vi "Camera.vi"(0 "Camera in":refnum<class "Camera.lvclass">, 1 "Stop":bool, 4 "BCG Image Processing":T2={"Brightness"=128.0, "Contrast"=45.0, "Gamma"=1.0} {"Brightness" scale=0.0..400.0; "Contrast" scale=0.0..90.0; "Gamma" scale=0.005..5.0}, 5 "error in (no error)":errorcluster, 6 "Machine Vision":T4, 7 "Camera settings":T1={"Gamma"=1.0, "Gain"=7, "Sharpness"=0, "Contrast"=0.009999999999999995, "Exposure"=0.0004073180282999787} {"Exposure" min=0.000244140625 max=0.5 scale=0.0002..0.5; "Contrast" min=0.0 max=1.0 scale=0.001..1.0; "Sharpness" min=0 max=2 step=1 scale=0.0..2.0; "Gain" min=0 max=100 step=1 scale=0.1..100.0; "Gamma" min=0.01 max=10.0 scale=0.01..10.0}, 10 "Material":T3, 12 "Loop 0":bool, 13 "Override presets":bool) -> (11 "Radius (Real-World)":dbl, 14 "Camera out":refnum<class "Camera.lvclass">, 15 "Average Strength":dbl, 17 "Image":T5(plugin-control), 18 "Camera":dbl[](array[numeric]), 19 "error out":errorcluster)   [LabVIEW 2018, in "Camera.lvclass"]
uses:
  Camera.lvclass
  Machine Vision.ctl
  Material.ctl
  Image processing.ctl
  Camera settings.ctl
  <vilib>/vision/NI_Vision_Development_Module.lvlib
panel:
  out "Y":sgl
  out "X":sgl
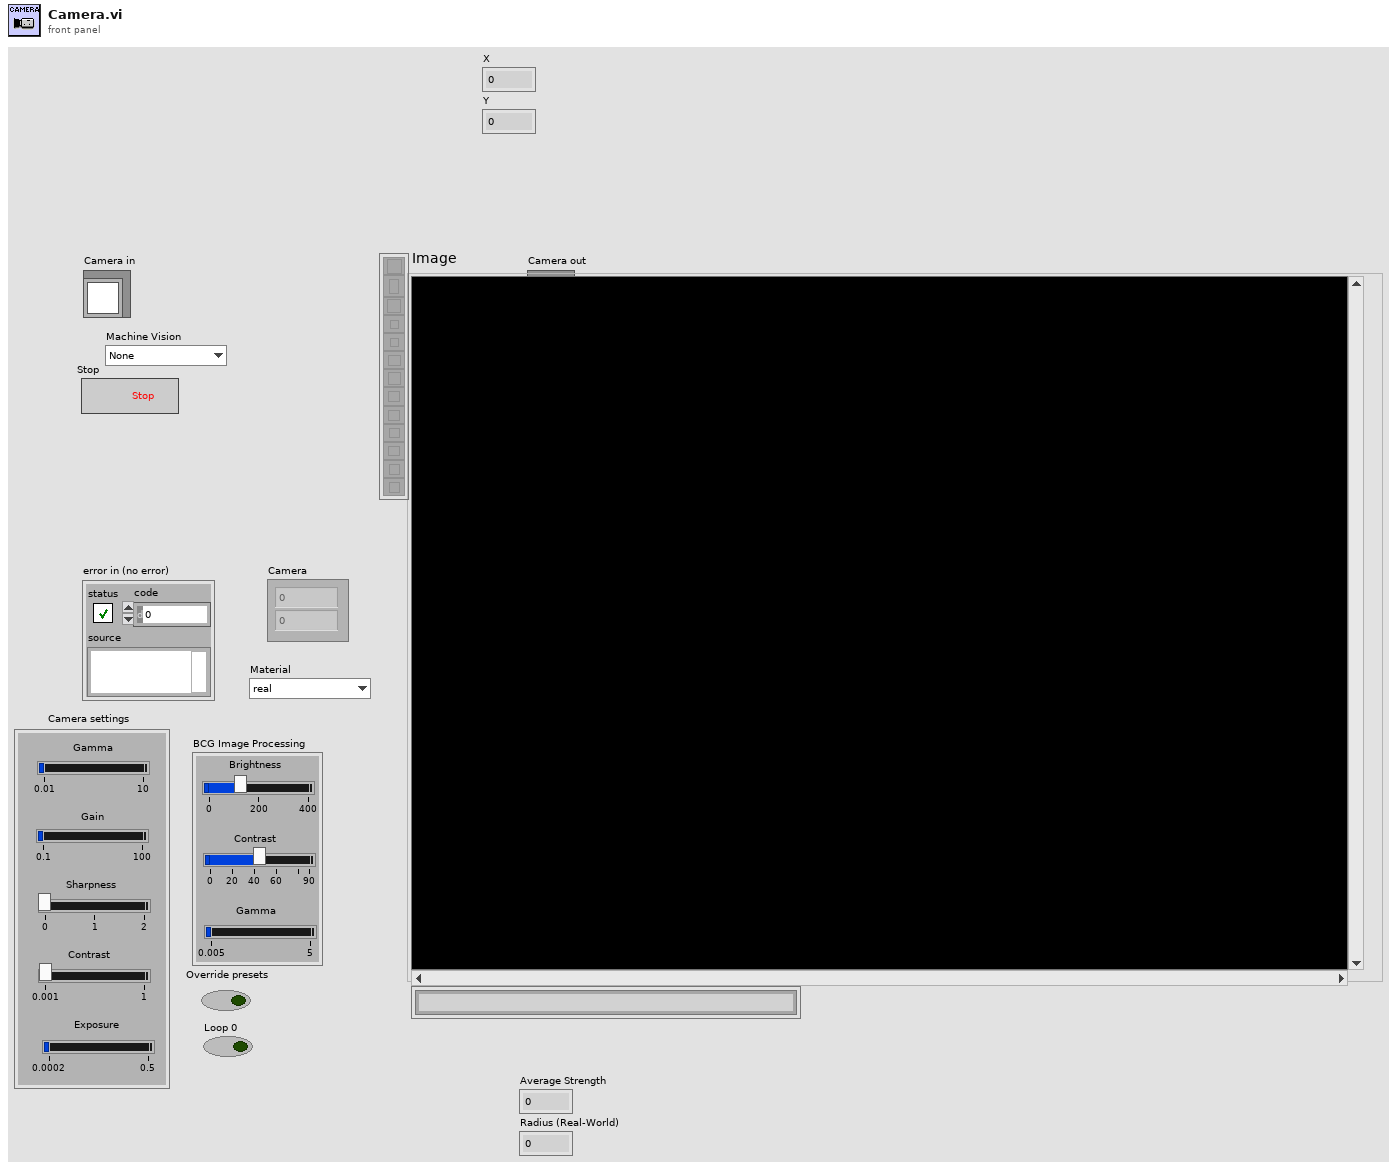
[diagram p1: front panel]
types:
  T1 = typedef "Camera.lvclass/Camera settings.ctl" = cluster{"Gamma":dbl, "Gain":i64, "Sharpness":i64, "Contrast":dbl, "Exposure":dbl}
  T2 = typedef "Camera.lvclass/Image processing.ctl" = cluster{"Brightness":sgl, "Contrast":sgl, "Gamma":sgl}
  T3 = typedef "Camera.lvclass/Material.ctl" = enum16{"real", "dummy", "PETG"}
  T4 = typedef "Camera.lvclass/Machine Vision.ctl" = enum16{"None", "Tray Fiducials", "HPK Silicon", "100um dot", "Hexaboard", "Corner (TL, BR)", "Corner (BL, TR)", "BP gold pad 1", "BP gold pad 2", "BP gold pad 3", "dummy sensor CH2", "dummy sensor CH7", "dummy sensor CH191", "dummy sensor CH197", "sensor box", "sensor circle", "PCB PETG CH2", "PCB PETG CH7", "PCB PETG CH191", "PCB PETG CH197"}
  T5 = typedef "IMAQ Image.ctl" = refnum<image>
  T6 = cluster{"Center (Pixels)":cluster{"X":sgl, "Y":sgl}, "Radius (Pixels)":dbl, "Center (Real-World)":cluster{"X":sgl, "Y":sgl}, "Radius (Real-World)":dbl, "Roundness (Real-World)":dbl, "Average Strength":dbl, "Average SNR (dB)":dbl}
  T7 = typedef "Edge New.ctl" = cluster{"Location (Pixel)":cluster{"X":sgl, "Y":sgl}, "Location (Real-World)":cluster{"X":sgl, "Y":sgl}, "Distance (Pixel)":dbl, "Distance (Real-World)":dbl, "Strength":dbl, "Noise":dbl, "Rising?":bool}
  T8 = cluster{"output string":sgl, "output string":sgl}
  T9 = typedef "ROI Descriptor" = cluster{"Global Rectangle":i32[], "Contours":cluster{"ID":enum32{"External", "Internal"}, "Type":u32, "Coordinates":i32[]}[]}
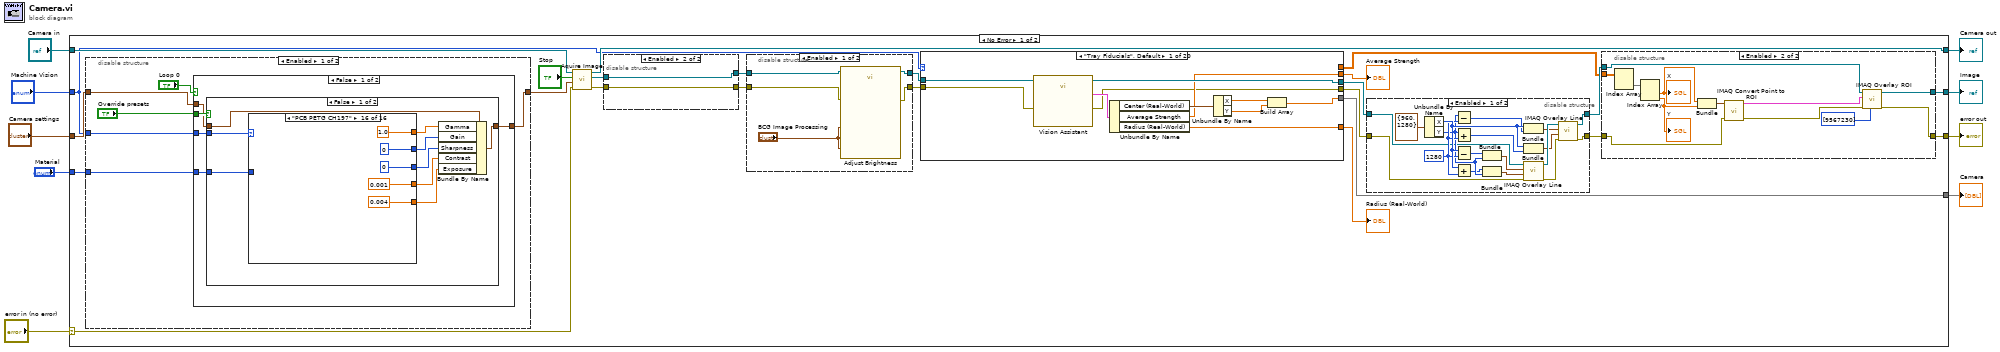
[diagram p0: block diagram]
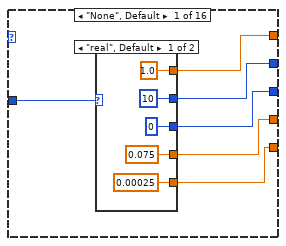
[diagram p5: hidden frame]
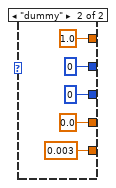
[diagram p6: hidden frame]
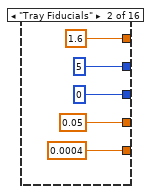
[diagram p7: hidden frame]
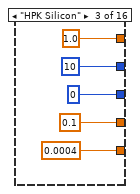
[diagram p8: hidden frame]
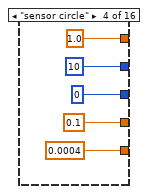
[diagram p9: hidden frame]
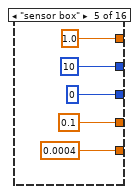
[diagram p10: hidden frame]
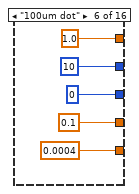
[diagram p11: hidden frame]
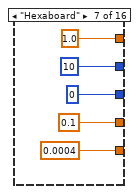
[diagram p12: hidden frame]
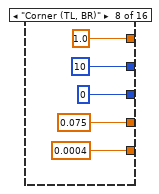
[diagram p13: hidden frame]
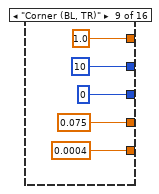
[diagram p14: hidden frame]
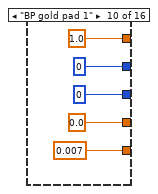
[diagram p15: hidden frame]
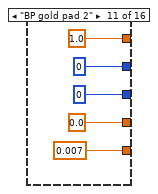
[diagram p16: hidden frame]
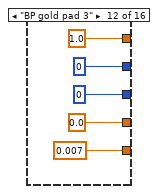
[diagram p17: hidden frame]
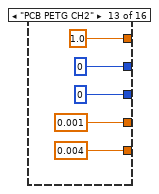
[diagram p18: hidden frame]
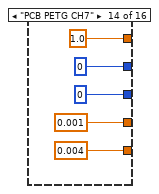
[diagram p19: hidden frame]
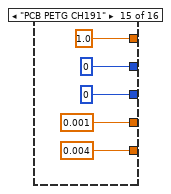
[diagram p20: hidden frame]
diagram:
  n1 = case shown="No Error" "error in (no error)" {
    selector: "error in (no error)" -> [w16 w391]
    tunnel: [w10 w391] -> w8
    tunnel: [w31 w390] -> w7
    tunnel: "Camera in" -> [w32 w390]
    tunnel: [w30 _] -> w5
    tunnel: [w20 _] -> w4
    tunnel: "Machine Vision" -> [w26 _]
    tunnel: "Camera settings" -> [w27 _]
    tunnel: "Material" -> [w25 _]
    frame No Error {
      n2 = disable-structure shown="Enabled" {
        disable-tunnel: w26 -> [w80 _]
        disable-tunnel: w27 -> [w79 w194]
        disable-tunnel: [w78 w194] -> w28
        disable-tunnel: w25 -> [w75 _]
        frame Enabled {
          n3 = case shown="False" "Loop 0" {
            tunnel: "Override presets" -> [w85 _]
            tunnel: w80 -> [w84 _]
            tunnel: w79 -> [w83 w193]
            tunnel: [w82 w192] -> w78
            tunnel: w75 -> [w81 _]
            frame False {
              n4 = case shown="False" w85 {
                tunnel: w84 -> [w94 _]
                tunnel: w83 -> [w93 w186]
                tunnel: [w87 w186] -> w82
                tunnel: w81 -> [w86 _]
                frame False {
                  n5 = case shown="\"PCB PETG CH197\"" w94 {
                    tunnel: [w99 1.6 ("Gamma::Value") 1.0 ("Gamma::Value") 1.0 ("Gamma::Value") 1.0 ("Gamma::Value") 1.0 ("Gamma::Value") 1.0 ("Gamma::Value") 1.0 ("Gamma::Value") 1.0 ("Gamma::Value") 1.0 ("Gamma::Value") 1.0 ("Gamma::Value") 1.0 ("Gamma::Value") 1.0 ("Gamma::Value") 1.0 ("Gamma::Value") 1.0 ("Gamma::Value") 1.0 ("Gamma::Value")] -> w92
                    tunnel: [w95 i64 5 ("Gain::Value") i64 10 ("Gain::Value") i64 10 ("Gain::Value") i64 10 ("Gain::Value") i64 10 ("Gain::Value") i64 10 ("Gain::Value") i64 10 ("Gain::Value") i64 10 ("Gain::Value") i64 0 ("Gain::Value") i64 0 ("Gain::Value") i64 0 ("Gain::Value") i64 0 ("Gain::Value") i64 0 ("Gain::Value") i64 0 ("Gain::Value") i64 0 ("Gain::Value")] -> w91
                    tunnel: [w96 i64 0 ("Sharpness::Value") i64 0 ("Sharpness::Value") i64 0 ("Sharpness::Value") i64 0 ("Sharpness::Value") i64 0 ("Sharpness::Value") i64 0 ("Sharpness::Value") i64 0 ("Sharpness::Value") i64 0 ("Sharpness::Value") i64 0 ("Sharpness::Value") i64 0 ("Sharpness::Value") i64 0 ("Sharpness::Value") i64 0 ("Sharpness::Value") i64 0 ("Sharpness::Value") i64 0 ("Sharpness::Value") i64 0 ("Sharpness::Value")] -> w90
                    tunnel: [w97 0.05 ("Contrast::Value") 0.1 ("Contrast::Value") 0.1 ("Contrast::Value") 0.1 ("Contrast::Value") 0.1 ("Contrast::Value") 0.1 ("Contrast::Value") 0.075 ("Contrast::Value") 0.075 ("Contrast::Value") 0.0 ("Contrast::Value") 0.0 ("Contrast::Value") 0.0 ("Contrast::Value") 0.001 ("Contrast::Value") 0.001 ("Contrast::Value") 0.001 ("Contrast::Value") 0.001 ("Contrast::Value")] -> w89
                    tunnel: [w98 0.0004 ("Exposure::Value") 0.0004 ("Exposure::Value") 0.0004 ("Exposure::Value") 0.0004 ("Exposure::Value") 0.0004 ("Exposure::Value") 0.0004 ("Exposure::Value") 0.0004 ("Exposure::Value") 0.0004 ("Exposure::Value") 0.007 ("Exposure::Value") 0.007 ("Exposure::Value") 0.007 ("Exposure::Value") 0.004 ("Exposure::Value") 0.004 ("Exposure::Value") 0.004 ("Exposure::Value") 0.004 ("Exposure::Value")] -> w88
                    tunnel: w86 -> [w100 _ _ _ _ _ _ _ _ _ _ _ _ _ _ _]
                    frame "None", Default {
                      n6 = case shown="\"real\", Default" w100 {
                        tunnel: [1.0 ("Gamma::Value") 1.0 ("Gamma::Value")] -> w99
                        tunnel: [0.00025 ("Exposure::Value") 0.003 ("Exposure::Value")] -> w98
                        tunnel: [0.075 ("Contrast::Value") 0.0 ("Contrast::Value")] -> w97
                        tunnel: [i64 0 ("Sharpness::Value") i64 0 ("Sharpness::Value")] -> w96
                        tunnel: [i64 10 ("Gain::Value") i64 0 ("Gain::Value")] -> w95
                        frame "real", Default {
                        }
                        frame "dummy" {
                        }
                      }
                    }
                    frame "Tray Fiducials" {
                    }
                    frame "HPK Silicon" {
                    }
                    frame "sensor circle" {
                    }
                    frame "sensor box" {
                    }
                    frame "100um dot" {
                    }
                    frame "Hexaboard" {
                    }
                    frame "Corner (TL, BR)" {
                    }
                    frame "Corner (BL, TR)" {
                    }
                    frame "BP gold pad 1" {
                    }
                    frame "BP gold pad 2" {
                    }
                    frame "BP gold pad 3" {
                    }
                    frame "PCB PETG CH2" {
                    }
                    frame "PCB PETG CH7" {
                    }
                    frame "PCB PETG CH191" {
                    }
                    frame "PCB PETG CH197" {
                    }
                  }
                  n7 = Bundle By Name(cluster=w93, "Gamma"=w92, "Gain"=w91, "Sharpness"=w90, "Contrast"=w89, "Exposure"=w88) -> (w87:T1)
                }
                frame True {
                }
              }
            }
            frame True {
              n8 = Bundle By Name(cluster=w193, "Gamma"=0.01, "Gain"=i64 0, "Sharpness"=i64 0, "Contrast"=0.0, "Exposure"=0.000249) -> (w192:T1)
            }
          }
        }
        frame Disabled {
        }
      }
      n9 = call-dynamic "Aquire Image.vi"("error in (no error)"=w16, "Cluster"=w28, "Stop"="Stop", "Camera in"=w32) -> ("error out"=w15:errorcluster, "Image Out"=w29:T5, "Camera out"=w31:refnum<class "Camera.lvclass">)  [unwired: 5 in]
      n10 = disable-structure shown="Enabled" {
        disable-tunnel: w29 -> [w201 w204]
        disable-tunnel: [w200 w204] -> w24
        disable-tunnel: w15 -> [w197 w203]
        disable-tunnel: [w195 w203] -> w14
        frame Disabled {
          w199 = u32 1 items=["Horizontal", "Vertical", "Central", "1st Diagonal", "2nd Diagonal"] ("Type of Symmetry")
          n11 = call "IMAQ Rotate"("error in (no error)"=w197, "Angle (degrees)"=270, "Image Src"=w201) -> ("error out"=w196:errorcluster, "Image Dst Out"=w198:T5)  [unwired: 7 in]
          n12 = call "IMAQ Symmetry"("error in (no error)"=w196, "Type of Symmetry"=w199, "Image Src"=w198) -> ("error out"=w195:errorcluster, "Image Dst Out"=w200:T5)  [unwired: 2 in]
        }
        frame Enabled {
        }
      }
      n13 = disable-structure shown="Enabled" {
        disable-tunnel: w24 -> [w72 w73]
        disable-tunnel: [w70 w73] -> w23
        disable-tunnel: w14 -> [w69 w74]
        disable-tunnel: [w68 w74] -> w13
        frame Enabled {
          n14 = call "Adjust Brightness"("Image In"=w72, "Red BCG Values (Brightness 1)"="BCG Image Processing", "Green BCG Values (Brightness 1)"="BCG Image Processing", "Blue BCG Values (Brightness 1)"="BCG Image Processing", "error in"=w69) -> ("Image Out"=w70:T5, "error out"=w68:errorcluster)  [unwired: 21 in]
        }
        frame Disabled {
        }
      }
      n15 = case shown="\"Tray Fiducials\", Default" w26 {
        tunnel: [w209 w219 w227 w238 w246 w254 w262 w270 w278 w287 w298 w304 w317 w323 w335 w347 w358 w366 w374 w382] -> w30
        tunnel: [w211 w221 w228 w240 w248 w256 w264 w272 w280 w288 w299 w310 w318 w327 w339 w351 w364 w372 w380 w388] -> w22
        tunnel: w23 -> [w212 w221 w226 w237 w245 w253 w261 w269 w277 w285 w296 w309 w315 w328 w340 w352 w365 w373 w381 w389]
        tunnel: [w207 0.0 ("Radius (Real-World)") w224 0.0 ("Radius (Real-World)") 0.0 ("Radius (Real-World)") 0.0 ("Radius (Real-World)") 0.0 ("Radius (Real-World)") 0.0 ("Radius (Real-World)") 0.0 ("Radius (Real-World)") w284 w295 0.0 ("Radius (Real-World)") w314 0.0 ("Radius (Real-World)") 0.0 ("Radius (Real-World)") 0.0 ("Radius (Real-World)") 0.0 ("Radius (Real-World)") 0.0 ("Radius (Real-World)") 0.0 ("Radius (Real-World)") 0.0 ("Radius (Real-World)")] -> w19
        tunnel: [w208 0.0 ("Strength") w225 _ _ _ _ _ _ w283 w294 _ w313 w333 w345 w357 _ _ _ _] -> w18
        tunnel: [_ _ _ w236 w244 w252 w260 w268 w276 _ _ w306 _ _ _ _ w360 w368 w376 w384] -> w17
        tunnel: w13 -> [w206 w220 w222 w235 w243 w249 w257 w265 w273 w282 w293 w308 w312 w326 w338 w350 w363 w371 w379 w387]
        tunnel: [w205 w220 w223 w234 w242 w250 w258 w266 w274 w281 w292 w307 w311 w325 w337 w349 w362 w370 w378 w386] -> w12
        frame "Tray Fiducials", Default {
          n16 = call "Vision Assistant"("Image In"=w212, "error in"=w206) -> ("Image Out"=w211:T5, "Fitted Circle (Find Circular Edge 1)"=w210:T6, "error out"=w205:errorcluster)  [unwired: 23 in]
          n17 = Unbundle By Name(w210) -> ("Center (Real-World)"=w213:cluster{"X":sgl, "Y":sgl}, "Average Strength"=w208:dbl, "Radius (Real-World)"=w207:dbl)
          n18 = Unbundle By Name(w213) -> ("X"=w215:sgl, "Y"=w214:sgl)
          n19 = Build Array(w215, w214) -> (w209:sgl[])
        }
        frame "None" {
          n20 = Initialize Array(0.0 ("element")) -> (w219:dbl[])  [unwired: 1 in]
        }
        frame "Hexaboard" {
          n21 = call "Vision Assistant2"("Image In"=w226, "error in"=w222) -> ("Image Out"=w228:T5, "Fitted Circle (Find Circular Edge 1)"=w230:T6, "error out"=w223:errorcluster)  [unwired: 23 in]
          n22 = Unbundle By Name(w230) -> ("Center (Real-World)"=w232:cluster{"X":sgl, "Y":sgl}, "Average Strength"=w225:dbl, "Radius (Real-World)"=w224:dbl)
          n23 = Unbundle By Name(w232) -> ("X"=w231:sgl, "Y"=w229:sgl)
          n24 = Build Array(w231, w229) -> (w227:sgl[])
        }
        frame "Corner (TL, BR)" {
          n25 = call "Vision Assistant3"("Image In"=w237, "error in"=w235) -> ("Image Out"=w240:T5, "error out"=w234:errorcluster, "Caliper Results (Top Left, Bottom Right)"=w236:sgl[][], "Calibrated Results (Top Left, Bottom Right)"=w239:sgl[][])  [unwired: 22 in]
          n26 = Index Array(array=w239) -> (element=w238:sgl[])  [unwired: 2 in]
        }
        frame "Corner (BL, TR)" {
          n27 = call "Vision Assistant4"("Image In"=w245, "error in"=w243) -> ("Image Out"=w248:T5, "error out"=w242:errorcluster, "Caliper Results (Bottom Left, Top Right)"=w244:sgl[][], "Calibrated Results (Bottom Left, Top Right)"=w247:sgl[][])  [unwired: 22 in]
          n28 = Index Array(array=w247) -> (element=w246:sgl[])  [unwired: 2 in]
        }
        frame "dummy sensor CH2" {
          n29 = call "Vision Assistant10"("Image In"=w253, "error in"=w249) -> ("Image Out"=w256:T5, "Caliper Results (Top Left, Bottom Right)"=w252:sgl[][], "Calibrated Results (Top Left, Bottom Right)"=w255:sgl[][], "error out"=w250:errorcluster)  [unwired: 22 in]
          n30 = Index Array(array=w255) -> (element=w254:sgl[])  [unwired: 2 in]
        }
        frame "dummy sensor CH7" {
          n31 = call "Vision Assistant11"("Image In"=w261, "error in"=w257) -> ("Image Out"=w264:T5, "Caliper Results (Top Left, Bottom Right)"=w260:sgl[][], "Calibrated Results (Top Left, Bottom Right)"=w263:sgl[][], "error out"=w258:errorcluster)  [unwired: 22 in]
          n32 = Index Array(array=w263) -> (element=w262:sgl[])  [unwired: 2 in]
        }
        frame "dummy sensor CH191" {
          n33 = call "Vision Assistant12"("Image In"=w269, "error in"=w265) -> ("Image Out"=w272:T5, "Caliper Results (Top Left, Bottom Right)"=w268:sgl[][], "Calibrated Results (Top Left, Bottom Right)"=w271:sgl[][], "error out"=w266:errorcluster)  [unwired: 22 in]
          n34 = Index Array(array=w271) -> (element=w270:sgl[])  [unwired: 2 in]
        }
        frame "dummy sensor CH197" {
          n35 = call "Vision Assistant13"("Image In"=w277, "error in"=w273) -> ("Image Out"=w280:T5, "Caliper Results (Top Left, Bottom Right)"=w276:sgl[][], "Calibrated Results (Top Left, Bottom Right)"=w279:sgl[][], "error out"=w274:errorcluster)  [unwired: 22 in]
          n36 = Index Array(array=w279) -> (element=w278:sgl[])  [unwired: 2 in]
        }
        frame "HPK Silicon" {
          n37 = call "Vision Assistant5"("Image In"=w285, "error in"=w282) -> ("Image Out"=w288:T5, "Fitted Circle (Find Circular Edge 1)"=w286:T6, "error out"=w281:errorcluster)  [unwired: 23 in]
          n38 = Unbundle By Name(w286) -> ("Center (Real-World)"=w291:cluster{"X":sgl, "Y":sgl}, "Average Strength"=w283:dbl, "Radius (Real-World)"=w284:dbl)
          n39 = Unbundle By Name(w291) -> ("X"=w290:sgl, "Y"=w289:sgl)
          n40 = Build Array(w290, w289) -> (w287:sgl[])
        }
        frame "sensor circle" {
          n41 = call "Vision Assistant14"("Image In"=w296, "error in"=w293) -> ("Image Out"=w299:T5, "Fitted Circle (Find Circular Edge 1)"=w297:T6, "error out"=w292:errorcluster)  [unwired: 23 in]
          n42 = Unbundle By Name(w297) -> ("Center (Real-World)"=w302:cluster{"X":sgl, "Y":sgl}, "Average Strength"=w294:dbl, "Radius (Real-World)"=w295:dbl)
          n43 = Unbundle By Name(w302) -> ("X"=w301:sgl, "Y"=w300:sgl)
          n44 = Build Array(w301, w300) -> (w298:sgl[])
        }
        frame "sensor box" {
          n45 = call "Vision Assistant15"("Image In"=w309, "error in"=w308) -> ("Image Out"=w310:T5, "Caliper Results (Caliper 1)"=w306:sgl[][], "Calibrated Results (Caliper 1)"=w305:sgl[][], "error out"=w307:errorcluster)  [unwired: 22 in]
          n46 = Index Array(array=w305) -> (element=w304:sgl[])  [unwired: 2 in]
        }
        frame "100um dot" {
          n47 = call "Vision Assistant6"("Image In"=w315, "error in"=w312) -> ("Image Out"=w318:T5, "Fitted Circle (Find Circular Edge 1)"=w316:T6, "error out"=w311:errorcluster)  [unwired: 23 in]
          n48 = Unbundle By Name(w316) -> ("Center (Real-World)"=w321:cluster{"X":sgl, "Y":sgl}, "Average Strength"=w313:dbl, "Radius (Real-World)"=w314:dbl)
          n49 = Unbundle By Name(w321) -> ("X"=w320:sgl, "Y"=w319:sgl)
          n50 = Build Array(w320, w319) -> (w317:sgl[])
        }
        frame "BP gold pad 1" {
          n51 = call "Vision Assistant7"("Image In"=w328, "error in"=w326) -> ("Image Out"=w327:T5, "Used Edges (Adv. Straight Edge 1)"=w332:cluster{"Edge Information":T7[]}[], "error out"=w325:errorcluster)  [unwired: 23 in]
          n52 = Index Array(array=w332) -> (element=w331:cluster{"Edge Information":T7[]})  [unwired: 1 in]
          n53 = Unbundle By Name(w331) -> ("Edge Information"=w330:T7[])
          n54 = Index Array(array=w330) -> (element=w329:T7)  [unwired: 1 in]
          n55 = Unbundle(w329) -> ("Location (Real-World)"=w324:cluster{"X":sgl, "Y":sgl}, "Strength"=w333:dbl)  [unwired: 5 out]
          n56 = Cluster To Array(cluster=w324) -> (array=w323:sgl[])
        }
        frame "BP gold pad 2" {
          n57 = call "Vision Assistant8"("Image In"=w340, "error in"=w338) -> ("Image Out"=w339:T5, "Used Edges (Adv. Straight Edge 1)"=w344:cluster{"Edge Information":T7[]}[], "error out"=w337:errorcluster)  [unwired: 23 in]
          n58 = Index Array(array=w344) -> (element=w343:cluster{"Edge Information":T7[]})  [unwired: 1 in]
          n59 = Unbundle By Name(w343) -> ("Edge Information"=w342:T7[])
          n60 = Index Array(array=w342) -> (element=w341:T7)  [unwired: 1 in]
          n61 = Unbundle(w341) -> ("Location (Real-World)"=w336:cluster{"X":sgl, "Y":sgl}, "Strength"=w345:dbl)  [unwired: 5 out]
          n62 = Cluster To Array(cluster=w336) -> (array=w335:sgl[])
        }
        frame "BP gold pad 3" {
          n63 = call "Vision Assistant9"("Image In"=w352, "error in"=w350) -> ("Image Out"=w351:T5, "Used Edges (Adv. Straight Edge 1)"=w356:cluster{"Edge Information":T7[]}[], "error out"=w349:errorcluster)  [unwired: 23 in]
          n64 = Index Array(array=w356) -> (element=w355:cluster{"Edge Information":T7[]})  [unwired: 1 in]
          n65 = Unbundle By Name(w355) -> ("Edge Information"=w354:T7[])
          n66 = Index Array(array=w354) -> (element=w353:T7)  [unwired: 1 in]
          n67 = Unbundle(w353) -> ("Location (Real-World)"=w348:cluster{"X":sgl, "Y":sgl}, "Strength"=w357:dbl)  [unwired: 5 out]
          n68 = Cluster To Array(cluster=w348) -> (array=w347:sgl[])
        }
        frame "PCB PETG CH2" {
          n69 = call "Vision Assistant16"("Image In"=w365, "error in"=w363) -> ("Image Out"=w364:T5, "Caliper Results (Caliper 1)"=w360:sgl[][], "Calibrated Results (Caliper 1)"=w359:sgl[][], "error out"=w362:errorcluster)  [unwired: 22 in]
          n70 = Index Array(array=w359) -> (element=w358:sgl[])  [unwired: 2 in]
        }
        frame "PCB PETG CH7" {
          n71 = call "Vision Assistant17"("Image In"=w373, "error in"=w371) -> ("Image Out"=w372:T5, "Caliper Results (Caliper 1)"=w368:sgl[][], "Calibrated Results (Caliper 1)"=w367:sgl[][], "error out"=w370:errorcluster)  [unwired: 22 in]
          n72 = Index Array(array=w367) -> (element=w366:sgl[])  [unwired: 2 in]
        }
        frame "PCB PETG CH191" {
          n73 = call "Vision Assistant18"("Image In"=w381, "error in"=w379) -> ("Image Out"=w380:T5, "Caliper Results (Caliper 1)"=w376:sgl[][], "Calibrated Results (Caliper 1)"=w375:sgl[][], "error out"=w378:errorcluster)  [unwired: 22 in]
          n74 = Index Array(array=w375) -> (element=w374:sgl[])  [unwired: 2 in]
        }
        frame "PCB PETG CH197" {
          n75 = call "Vision Assistant19"("Image In"=w389, "error in"=w387) -> ("Image Out"=w388:T5, "Caliper Results (Caliper 1)"=w384:sgl[][], "Calibrated Results (Caliper 1)"=w383:sgl[][], "error out"=w386:errorcluster)  [unwired: 22 in]
          n76 = Index Array(array=w383) -> (element=w382:sgl[])  [unwired: 2 in]
        }
      }
      "Radius (Real-World)" <- w19
      "Average Strength" <- w18
      n77 = disable-structure shown="Enabled" {
        disable-tunnel: w22 -> [w52 w67]
        disable-tunnel: [w51 w67] -> w21
        disable-tunnel: w12 -> [w50 w66]
        disable-tunnel: [w48 w66] -> w11
        frame Enabled {
          w59 = 1280
          n78 = Unbundle By Name(cluster{"X":i32, "Y":i32} {"X"=960, "Y"=1280} ("Cross Hair coordinates")) -> ("X"=w62:i32, "Y"=w58:i32)
          n79 = Subtract(x=w58, y=w59) -> (x-y=w60:i32)
          n80 = Add(x=w58, y=w59) -> (x+y=w61:i32)
          n81 = Subtract(x=w62, y=w59) -> (x-y=w54:i32)
          n82 = Add(x=w62, y=w59) -> (x+y=w55:i32)
          n83 = Bundle(w54, "Y"=w58) -> (w57:cluster{i32, "Y":i32})  [unwired: 1 in]
          n84 = Bundle(w55, "Y"=w58) -> (w56:cluster{i32, "Y":i32})  [unwired: 1 in]
          n85 = Bundle("X"=w62, w60) -> (w63:cluster{"X":i32, i32})  [unwired: 1 in]
          n86 = Bundle("X"=w62, w61) -> (w64:cluster{"X":i32, i32})  [unwired: 1 in]
          n87 = call "IMAQ Overlay Line"("error in (no error)"=w50, "End Point"=w56, "Start Point"=w57, "Image"=w52) -> ("error out"=w49:errorcluster, "Image Out"=w65:T5)  [unwired: 6 in]
          n88 = call "IMAQ Overlay Line"("error in (no error)"=w49, "End Point"=w64, "Start Point"=w63, "Image"=w65) -> ("error out"=w48:errorcluster, "Image Out"=w51:T5)  [unwired: 6 in]
        }
        frame Disabled {
        }
      }
      n89 = disable-structure shown="Enabled" {
        disable-tunnel: [w35 w43] -> w20
        disable-tunnel: w21 -> [w35 w42]
        disable-tunnel: w17 -> [_ w41]
        disable-tunnel: w11 -> [w34 w38]
        disable-tunnel: [w34 w36] -> w10
        frame Disabled {
        }
        frame Enabled {
          n90 = Index Array(array=w41) -> (element=w40:sgl[])  [unwired: 2 in]
          n91 = Index Array(array=w40) -> (element #1=w44:sgl, element #2=w46:sgl)  [unwired: 2 in]
          "X" <- w44
          "Y" <- w46
          n92 = Bundle("output string"=w44, "output string"=w46) -> (w47:T8)  [unwired: 1 in]
          n93 = call "IMAQ Convert Point to ROI"("error in (no error)"=w38, "Point"=w47) -> ("error out"=w37:errorcluster, "ROI Descriptor"=w45:T9)  [unwired: 7 in]
          n94 = call "IMAQ Overlay ROI"("Colors (Green)"=u32[] [9567230], "error in (no error)"=w37, "ROI Descriptor"=w45, "Image"=w42) -> ("error out"=w36:errorcluster, "Image Out"=w43:T5)  [unwired: 6 in]
        }
      }
    }
    frame Error {
    }
  }
  "error out" <- w8
  "Camera out" <- w7
  "Camera" <- w5
  "Image" <- w4
